vi "camera_selector.vi"(1 "IMAQ interface name":string="img0", 2 "Use external trigger for camera control (IMAQ only)":bool) -> (0 "output cluster":T2)   [LabVIEW 2015]
uses:
  <vilib>/userdefined/High Color/IMAQdx.ctl
  <vilib>/vision/Avi1.llb/AviRefnum.ctl
  <vilib>/vision/driver/NI_Vision_Acquisition_Software.lvlib
panel:
  out "Avi Refnum":T3
  out "IMAQ Session Out":refnum<k11>
  in  "AVI Path":path
  in  "IMAQdx Session":T1="cam0"
  in  "Accept":bool
  in  "Stop":bool
  in  "Image Data Input Source":T4(radio)
  out "error out":errorcluster
  out "IMAQ error":errorcluster
  # "Multi-Worm Tracker \n\n            Image Input Source Selector"
  # "(CameraLink)"
  # "(USB,FireWire, GigE)"
  # "(Pre-recorded)"
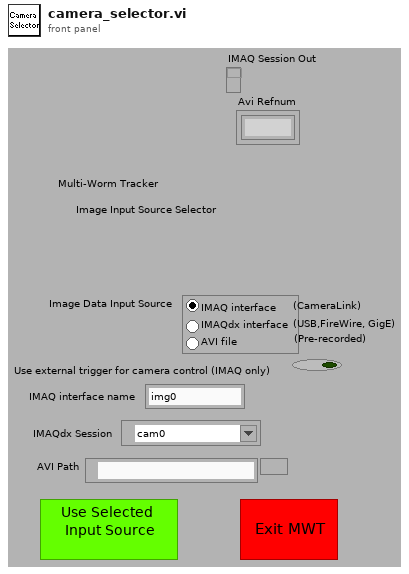
[diagram p1: front panel]
types:
  T1 = typedef "IMAQdx.ctl" = refnum<k21>
  T2 = cluster{"Value":refnum<k11>, "Value":refnum<k1>, "Value":enum32{"IMAQ interface", "IMAQdx interface", "AVI file"}, cluster{"Value":string, "Value":T1, "Value":path}, bool, "Value":bool}
  T3 = typedef "AviRefnum.ctl" = refnum<k1>
  T4 = enum32{"IMAQ interface", "IMAQdx interface", "AVI file"}
  T5 = cluster{"Value":string, "Value":T1, "Value":path}
  T6 = cluster{"Value":refnum<k11>, "Value":T3, "Value":enum32{"IMAQ interface", "IMAQdx interface", "AVI file"}, cluster{"Value":string, "Value":T1, "Value":path}, bool, "Value":bool}
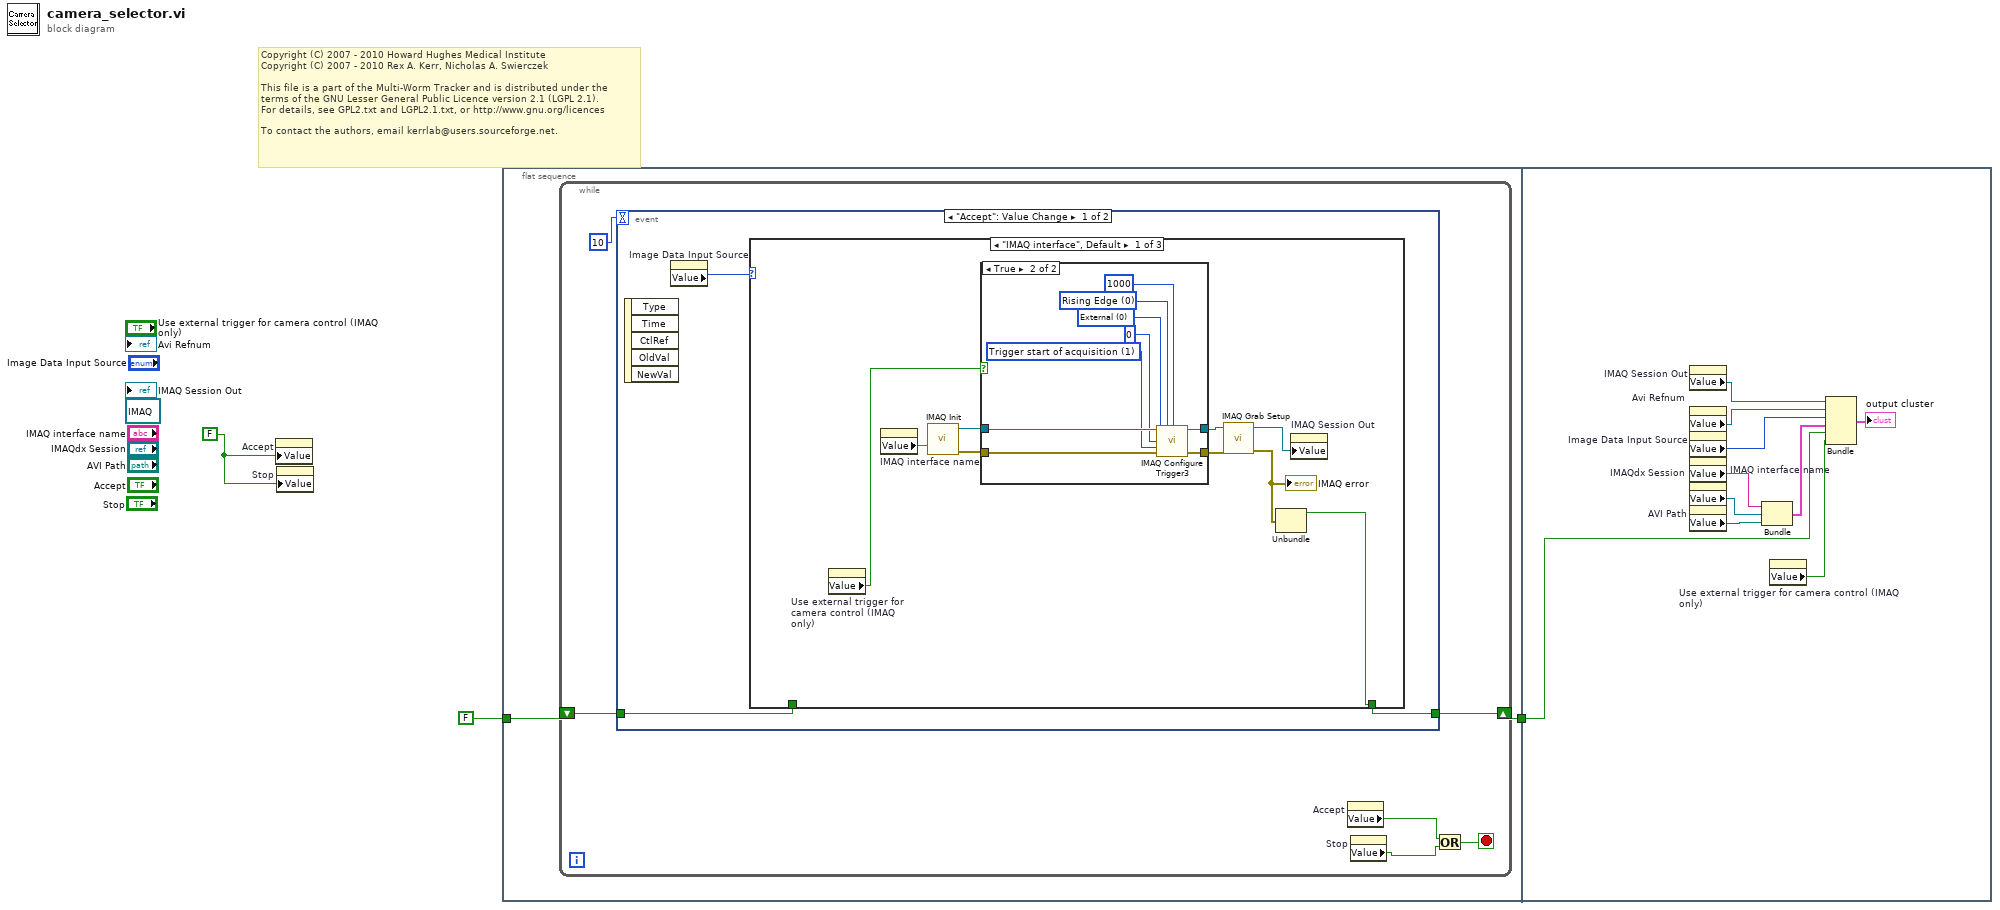
[diagram p0: block diagram]
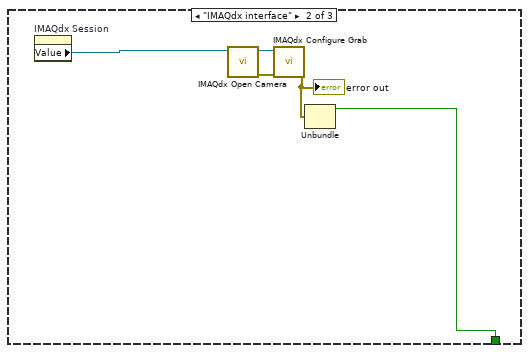
[diagram p3: hidden frame]
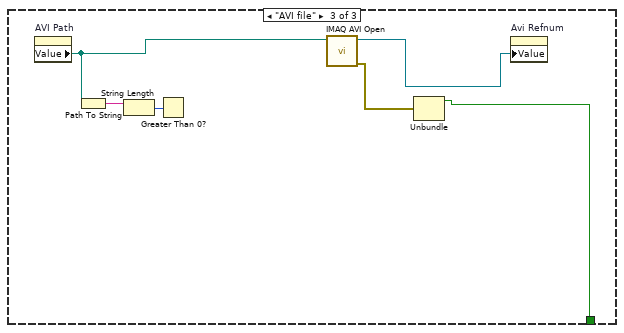
[diagram p4: hidden frame]
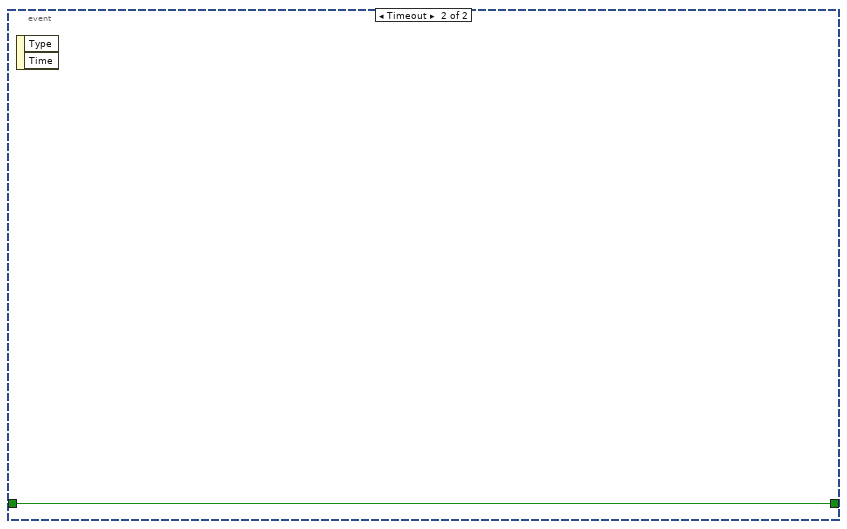
[diagram p5: hidden frame]
diagram:
  w2 = FALSE
  (unwired) refnum<k11> refnum ("IMAQ Session Out")
  # "Copyright (C) 2007 - 2010 Howard Hughes Medical Institute\nCopyright (C) 2007 - 2010 Rex A. Kerr, Nicholas A. Swierczek\n \nThis file is a part of the Multi-Worm Tracker and is distributed under the\nterms of the GNU Lesser General Public Licence version 2.1 (LGPL 2.1).\nFor details, see GPL2.txt and LGPL2.1.txt, or http://www.gnu.org/licences\n \nTo contact the authors, email kerrlab@users.sourceforge.net."
  n1 = property on="Accept" class="Bool (strict)"("Value"=w2) -> ()  [unwired: 2 in, 2 out]
  n2 = property on="Stop" class="Bool (strict)"("Value"=w2) -> ()  [unwired: 2 in, 2 out]
  n3 = flat-sequence {
    tunnel: FALSE -> [w5]
    tunnel: [w4] -> w1
    tunnel: w1 -> [w53]
    frame #0 {
      n4 = while {
        shift-right: [w11] -> w4
        shift-left: w5 -> [w10]
        stop <- w6 stop-if-true
        n5 = event shown="[0] \"Accept\": Value Change" {
          selector: _ -> [_ _]
          dyn-events: _ -> [_ _]
          timeout: 10 -> [_ _]
          tunnel: [w14 w46] -> w11
          tunnel: w10 -> [w13 w46]
          event "Accept": Value Change {
            n6 = event-data() -> ()  [unwired: 1 in, 5 out]
            n7 = property on="Image Data Input Source" class="RadioBtnsControl (strict)"() -> ("Value"=w12:T4)  [unwired: 2 in, 2 out]
            n8 = case shown="\"IMAQ interface\", Default" w12 {
              tunnel: [w23 w39 w45] -> w14
              tunnel: w13 -> [_ _ _]
              frame "IMAQ interface", Default {
                n9 = property on="Use external trigger for camera control (IMAQ only)" class="Bool (strict)"() -> ("Value"=w21:bool)  [unwired: 2 in, 2 out]
                n10 = property on="IMAQ interface name" class="Str"() -> ("Value"=w22:string)  [unwired: 2 in, 2 out]
                n11 = call <vilib>:"IMAQ Init.vi"("Interface Name"=w22) -> ("error out"=w19:errorcluster, "IMAQ Session Out"=w20:refnum<k11>)  [unwired: 9 in]
                n12 = case shown="True" w21 {
                  tunnel: w20 -> [w25 w34]
                  tunnel: [w25 w33] -> w18
                  tunnel: w19 -> [w24 w32]
                  tunnel: [w24 w31] -> w17
                  frame False {
                  }
                  frame True {
                    w26 = u32 1 items=["Disabled", "Trigger start of acquisition", "Trigger start of each buffer list", "Trigger each buffer", "Trigger each line (linescan)", "Trigger end of acquisition"] ("Action")
                    w28 = u32 0 items=["External"=0, "RTSI"=1, "ISO In"=2, "Scaled Encoder"=5, "Software Trigger"=6] ("Type")
                    w29 = u32 0 items=["Rising Edge", "Falling Edge"] ("Polarity")
                    n13 = call <vilib>:"IMAQ Configure Trigger3.vi"("IMAQ Session In"=w34, "Polarity"=w29, "Frame timeout (ms)"=u32 1000, "Type"=w28, "Line Number"=u32 0, "Action"=w26, "error in (no error)"=w32) -> ("IMAQ Session Out"=w33:refnum<k11>, "error out"=w31:errorcluster)  [unwired: 7 in]
                  }
                }
                n14 = call <vilib>:"IMAQ Grab Setup.vi"("error in (no error)"=w17, "IMAQ Session In"=w18) -> ("error out"=w15:errorcluster, "IMAQ Session Out"=w16:refnum<k11>)  [unwired: 8 in]
                "IMAQ error" <- w15
                n15 = Unbundle(w15) -> ("status"=w23:bool)  [unwired: 2 out]
                n16 = property on="IMAQ Session Out" class="Ref (strict)"("Value"=w16) -> ()  [unwired: 2 in, 2 out]
              }
              frame "IMAQdx interface" {
                n17 = property on="IMAQdx Session" class="IMAQdx (strict)"() -> ("Value"=w35:T1)  [unwired: 2 in, 2 out]
                n18 = call <vilib>:"IMAQdx Open Camera.vi"("Session In"=w35) -> ("error out"=w38:errorcluster, "Session Out"=w37:T1)  [unwired: 9 in]
                n19 = call <vilib>:"IMAQdx Configure Grab.vi"("error in"=w38, "Session In"=w37) -> ("error out"=w36:errorcluster)  [unwired: 8 in, 1 out]
                "error out" <- w36
                n20 = Unbundle(w36) -> ("status"=w39:bool)  [unwired: 2 out]
              }
              frame "AVI file" {
                n21 = property on="AVI Path" class="Path"() -> ("Value"=w44:path)  [unwired: 2 in, 2 out]
                n22 = Path To String(path=w44) -> (string=w43:string)
                n23 = String Length(string=w43) -> (length=w42:i32)
                n24 = Greater Than 0?(x=w42) -> ()  [unwired: 1 out]
                n25 = call "IMAQ AVI Open"("AVI Path"=w44) -> ("error out"=w40:errorcluster, "Avi Refnum"=w41:T3)  [unwired: 9 in]
                n26 = Unbundle(w40) -> ("status"=w45:bool)  [unwired: 2 out]
                n27 = property on="Avi Refnum" class="TypRef (strict)"("Value"=w41) -> ()  [unwired: 2 in, 2 out]
              }
            }
          }
          event Timeout {
            n28 = event-data() -> ()  [unwired: 1 in, 2 out]
          }
        }
        n29 = property on="Accept" class="Bool (strict)"() -> ("Value"=w9:bool)  [unwired: 2 in, 2 out]
        n30 = property on="Stop" class="Bool (strict)"() -> ("Value"=w8:bool)  [unwired: 2 in, 2 out]
        n31 = Or(x=w9, y=w8) -> (x .or. y?=w6:bool)
      }
    }
    frame #1 {
      n32 = property on="IMAQ Session Out" class="Ref (strict)"() -> ("Value"=w50:refnum<k11>)  [unwired: 2 in, 2 out]
      n33 = property on="Avi Refnum" class="TypRef (strict)"() -> ("Value"=w49:T3)  [unwired: 2 in, 2 out]
      n34 = property on="Image Data Input Source" class="RadioBtnsControl (strict)"() -> ("Value"=w56:T4)  [unwired: 2 in, 2 out]
      n35 = property on="IMAQ interface name" class="Str"() -> ("Value"=w55:string)  [unwired: 2 in, 2 out]
      n36 = property on="IMAQdx Session" class="IMAQdx (strict)"() -> ("Value"=w51:T1)  [unwired: 2 in, 2 out]
      n37 = property on="AVI Path" class="Path"() -> ("Value"=w52:path)  [unwired: 2 in, 2 out]
      n38 = Bundle("Value"=w55, "Value"=w51, "Value"=w52) -> (w54:T5)  [unwired: 1 in]
      n39 = property on="Use external trigger for camera control (IMAQ only)" class="Bool (strict)"() -> ("Value"=w48:bool)  [unwired: 2 in, 2 out]
      n40 = Bundle("Value"=w50, "Value"=w49, "Value"=w56, w54, w53, "Value"=w48) -> (→"output cluster":T6)  [unwired: 1 in]
    }
  }
